vi "ASCIIToUTF8.vi"(8 "error in":errorcluster, 11 "LV Text":string) -> (0 "error out":errorcluster, 3 "UTF-8 Text":string)   [LabVIEW 2020, in "Other.lvlib"]
uses:
  Other.lvlib
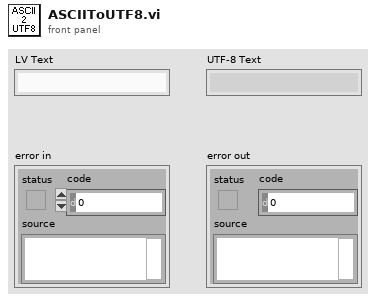
[diagram p1: front panel]
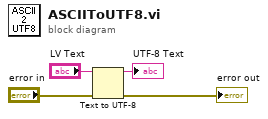
[diagram p0: block diagram]
diagram:
  n1 = Text to UTF-8(8:"error in", 11:"LV Text") -> (0:→"error out":errorcluster, 3:→"UTF-8 Text":string)  [unwired: 1 in]
